vi "testtest.vi"() -> ()   [LabVIEW 2017]
uses:
  <vilib>/Utility/file.llb/Read Delimited Spreadsheet (DBL).vi
panel:
  out "subarray":dbl[](array[numeric])
  out "Numeric":dbl
  out "length":i32
  out "index":i32
  out "Numeric 2":dbl
  in  "file path (dialog if empty) 3":path
  out "all rows 3":dbl[][](array[numeric])
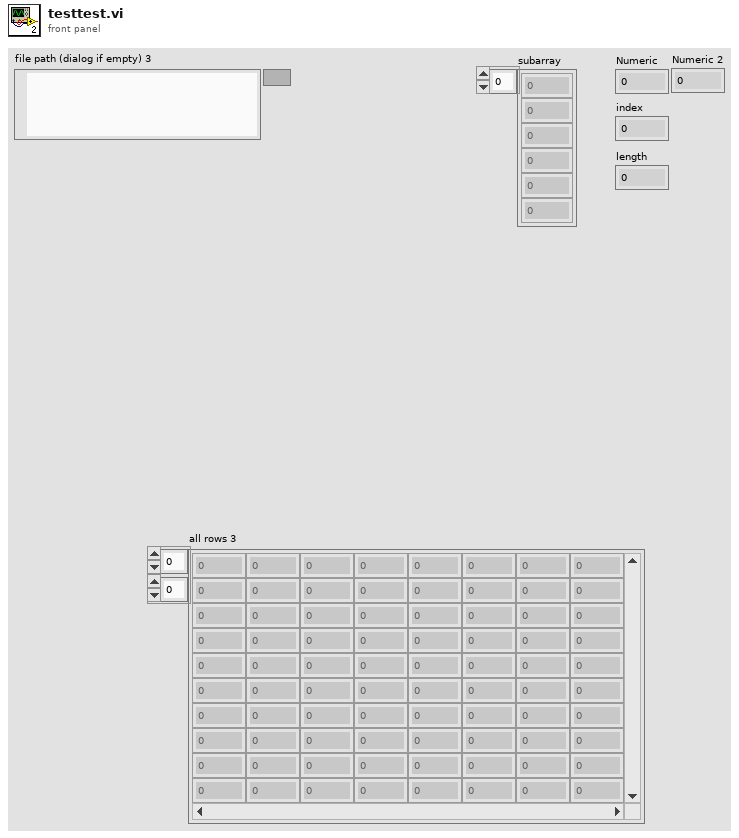
[diagram p1: front panel]
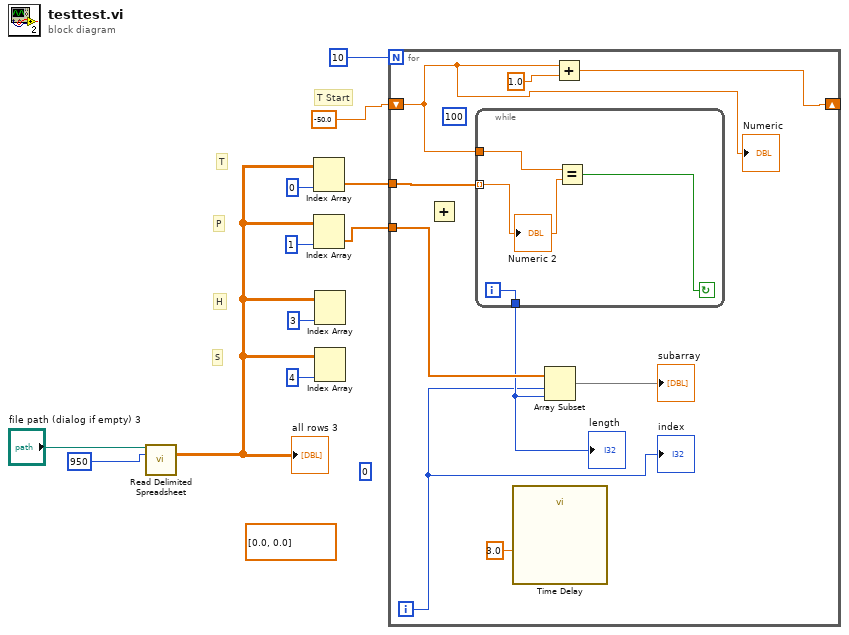
[diagram p0: block diagram]
diagram:
  (unwired) 0 ("number of rows (all:-1)")
  (unwired) dbl[][] [[0.0], [0.0]]
  # "T Start"
  # "S"
  # "H"
  # "P"
  # "T"
  n1 = call-poly <vilib>:"Read Delimited Spreadsheet.vi"("file path (dialog if empty)"="file path (dialog if empty) 3", "number of rows (all:-1)"=950) -> ("all rows"=w5:dbl[][])  [unwired: 8 in, 5 out]
  "all rows 3" <- w5
  n2 = Index Array(array=w5, index (col)=0 ("disabled index (col)")) -> (element=w4:dbl[])  [unwired: 1 in]
  n3 = Index Array(array=w5, index (col)=1) -> (element=w2:dbl[])  [unwired: 1 in]
  n4 = Index Array(array=w5, index (col)=3 ("disabled index (col)")) -> ()  [unwired: 1 in, 1 out]
  n5 = Index Array(array=w5, index (col)=4) -> ()  [unwired: 1 in, 1 out]
  n6 = for {
    N: 10 ("number of rows (all:-1)") -> [_]
    tunnel: w4 -> [w20]
    shift-right: [w18] -> _
    shift-left: -50.0 ("Numeric") -> [w14]
    tunnel: w2 -> [w17]
    i -> [w12]
    (unwired) 100
    n7 = Add() -> ()  [unwired: 2 in, 1 out]
    n8 = while {
      tunnel: w20 -> [w24] mode=indexing
      tunnel: [w23] -> w13
      tunnel: w14 -> [w22]
      i -> [w23]
      stop <- w21 continue-if-true
      n9 = Equal?(x=w22, y=w24) -> (x = y?=w21:bool)
      "Numeric 2" <- w24
    }
    "length" <- w13
    n10 = call "Time Delay"("Delay Time (s)"=3.0) -> ()  [unwired: 10 in, 1 out]
    n11 = Array Subset(array=w17, index=w12, length=w13) -> (→"subarray":dbl[])
    n12 = Add(x=w14, y=1.0) -> (x+y=w18:dbl)
    "Numeric" <- w14
    "index" <- w12
  }
